vi "PH_AxisGUI_NF.set i Attr.vi"(2 "error in (no error)":errorcluster, 3 "DB Entry to read":string) -> (0 "error out":errorcluster, 1 "i Attributes":T1={"GUI Refs"={"Delete"=refnum, "Slide 0"=refnum, "Slide 1"=refnum, "Slide 2"=refnum, "Instance Status"=refnum, "Position"=refnum, "Reset"=refnum, "Goal"=refnum, "Go"=refnum}, "Instance"="N/A", "Name Axis 0"="N/A", "Name Axis 1"="N/A", "Name Axis 2"="N/A", "System"="N/A", "Driver Type"=enum."not defined", "Offset"=0, "Goal"=0})   [LabVIEW 2014, in "PH_AxisGUI_NF.lvlib"]
doc: "This VI reads the DB entries and sets several attributes and GUI element settings."
uses:
  PH_AxisGUI_NF.lvlib
  PH_AxisGUI_NF.i attribute.ctl
  CS_Motion/NF87XX/NF87XX.driver Type.ctl
  CS_Motion/NF87XX/NF87XX.lvlib
  PH_Basics/PH_Common/PH_Common.lvlib
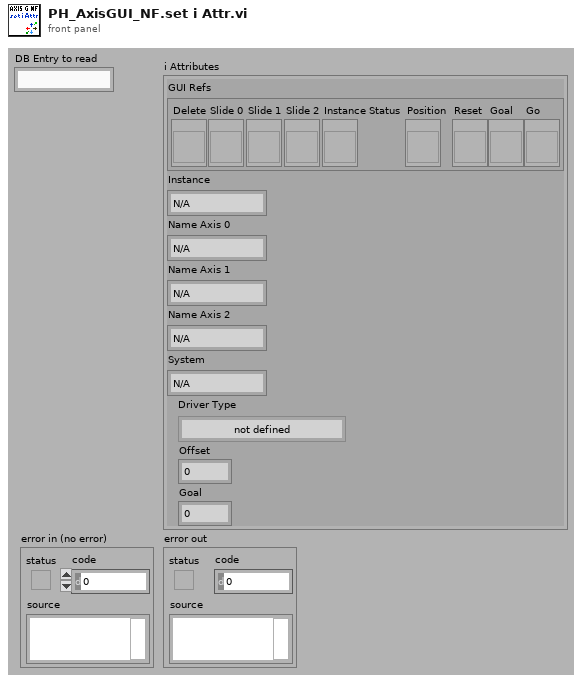
[diagram p1: front panel]
types:
  T1 = typedef "PH_AxisGUI_NF.lvlib/PH_AxisGUI_NF.i attribute.ctl" = cluster{"GUI Refs":cluster{"Delete":refnum<vi>, "Slide 0":refnum<vi>, "Slide 1":refnum<vi>, "Slide 2":refnum<vi>, "Instance Status":refnum<vi>, "Position":refnum<vi>, "Reset":refnum<vi>, "Goal":refnum<vi>, "Go":refnum<vi>}, "Instance":string, "Name Axis 0":string, "Name Axis 1":string, "Name Axis 2":string, "System":string, "Driver Type":T2, "Offset":i32, "Goal":i32}
  T2 = typedef "NF87XX.lvlib/NF87XX.driver Type.ctl" = enum16{"not defined", "3-ch open loop drv", "1-ch closed loop drv"}
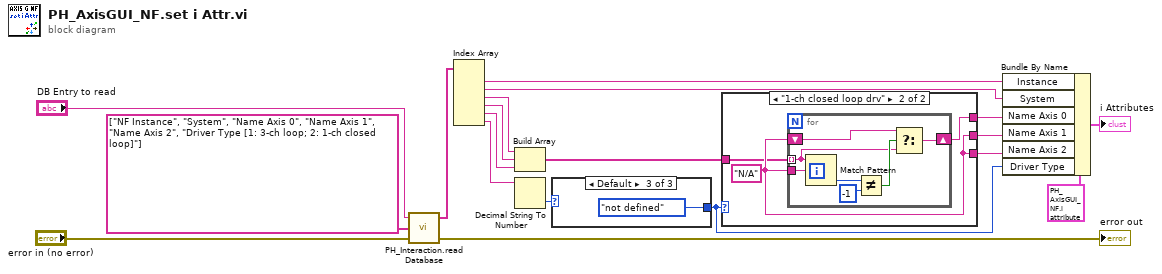
[diagram p0: block diagram]
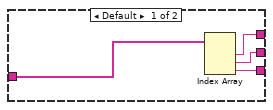
[diagram p2: hidden frame]
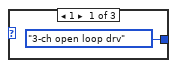
[diagram p3: hidden frame]
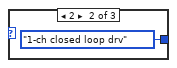
[diagram p4: hidden frame]
diagram:
  n1 = call "PH_Interaction.read Database.vi"("error in (no error)"="error in (no error)", "Strings to search for"=string[] ["NF Instance", "System", "Name Axis 0", "Name Axis 1", "Name Axis 2", "Driver Type [1: 3-ch loop; 2: 1-ch closed loop]"], "DB Entry to read"="DB Entry to read") -> ("error out"=→"error out":errorcluster, "Values"=w8:string[])  [unwired: 1 in]
  n2 = Index Array(array=w8) -> (element #1=w18:string, element #2=w17:string, element #3=w6:string, element #4=w5:string, element #5=w4:string, element #6=w7:string)  [unwired: 6 in]
  n3 = Build Array(w6, w5, w4) -> (w3:string[])
  n4 = Decimal String To Number(string=w7) -> (number=w16:i32)  [unwired: 2 in, 1 out]
  n5 = case shown="Default" w16 {
    tunnel: [NF87XX.driver_Type."3-ch open loop drv" ("Driver Type") NF87XX.driver_Type."1-ch closed loop drv" ("Driver Type") NF87XX.driver_Type."not defined" ("Driver Type")] -> w1
    frame 1 {
    }
    frame 2 {
    }
    frame Default {
    }
  }
  n6 = case shown="\"1-ch closed loop drv\"" w1 {
    tunnel: [w25 w29] -> w15
    tunnel: [w24 w29] -> w14
    tunnel: [w26 w28] -> w13
    tunnel: w3 -> [w23 w27]
    frame Default {
      n7 = Index Array(array=w23) -> (element #1=w26:string, element #2=w24:string, element #3=w25:string)  [unwired: 3 in]
    }
    frame "1-ch closed loop drv" {
      w29 = "N/A"
      n8 = for {
        tunnel: w27 -> [w30] mode=indexing
        tunnel: w29 -> [w36]
        shift-right: [w31] -> w28
        shift-left: w29 -> [w32]
        n9 = Match Pattern(string=w30, regular expression=w36) -> (offset past match=w35:i32)  [unwired: 1 in, 3 out]
        n10 = Not Equal?(x=w35, y=-1) -> (x != y?=w33:bool)
        n11 = Select(t=w32, s=w33, f=w30) -> (s? t:f=w31:string)
      }
    }
  }
  n12 = Bundle By Name(cluster=T1 {"GUI Refs"={"Delete"=refnum, "Slide 0"=refnum, "Slide 1"=refnum, "Slide 2"=refnum, "Instance Status"=refnum, "Position"=refnum, "Reset"=refnum, "Goal"=refnum, "Go"=refnum}, "Instance"="N/A", "Name Axis 0"="N/A", "Name Axis 1"="N/A", "Name Axis 2"="N/A", "System"="N/A", "Driver Type"=enum."not defined", "Offset"=0, "Goal"=0} ("i attribute"), "Instance"=w18, "System"=w17, "Name Axis 0"=w13, "Name Axis 1"=w14, "Name Axis 2"=w15, "Driver Type"=w1) -> (→"i Attributes":T1)
